vi "tx.vi"(1 "Modulation Parameters In":T2 {"TX Parameters"."TX Sample Rate" items=["4M"]}, 3 "HW parameters in":T3={"Device IP Address"="192.168.11.3", "Active Antenna"="RF1", "Carrier Frequency (Hz)"=2400000000.0, "Gain (dB)"=10.0, "Generation Mode"=enum."single shot"} {"Gain (dB)" format="%.2f"; "Carrier Frequency (Hz)" format="%.2p"}, 5 "Queues in":T1, 7 "error in":errorcluster, 8 "Symbol Energy":dbl=1.0 format="%#_4p") -> (9 "Transmitted IQ Graph":cluster{dbl[], dbl[]}(graph) caption="IQ Graph", 10 "Transmitted Magnitude":dbl[](graph), 11 "Transmitted Constellation Graph":T5(graph) caption="Constellation Graph", 13 "Transmitted Eye Diagram":cluster{"t0":dbl, "dt":dbl, "Y":dbl[]}[](graph) caption="Eye Diagram", 15 "Transmitted I":waveform(dbl)(graph), 16 "Transmitted Phase":dbl[](graph), 17 "Transmitted Q":waveform(dbl)(graph), 19 "Transmitted PSD":dbl[](graph), 20 "HW parameters out":T3={"Device IP Address"="192.168.11.3", "Active Antenna"="RF1", "Carrier Frequency (Hz)"=2400000000.0, "Gain (dB)"=10.0, "Generation Mode"=enum."single shot"} {"Gain (dB)" format="%.2f"; "Carrier Frequency (Hz)" format="%.2p"}, 21 "output complex waveform":cluster{"t0":dbl, "dt":dbl, "Y":cdb[]}, 23 "key bit sequence":u8[](array[numeric]), 25 "data symbols":cdb[](array[numeric]), 27 "error out":errorcluster)   [LabVIEW 2012]
uses:
  EE 497/LABS/SDR/control_type_defs.llb/tx_hw params.ctl
  EE 497/LABS/SDR/control_type_defs.llb/Queues.ctl
panel:
  out "number of data symbols":i32
  in  "TX Graphs":T4(tab)
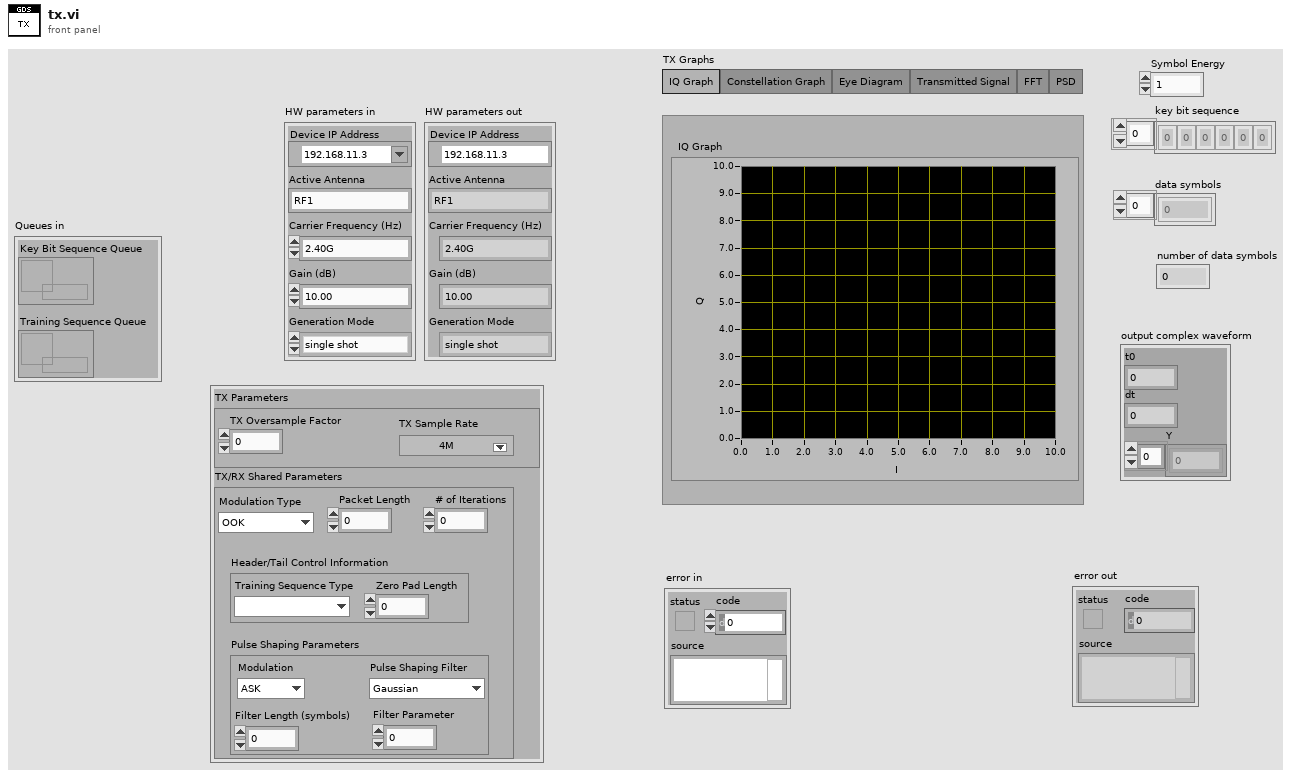
[diagram p1: front panel]
types:
  T1 = typedef "Queues.ctl" = cluster{"Key Bit Sequence Queue":refnum<queue>, "Training Sequence Queue":refnum<queue>}
  T2 = cluster{"TX Parameters":cluster{"TX Oversample Factor":u16, "TX Sample Rate":dbl}, "TX/RX Shared Parameters":cluster{"Modulation Type":enum16{"OOK", "FSK"}, "Packet Length":dbl, "# of Iterations":dbl, "Pulse Shaping Parameters":cluster{"Modulation":enum16{"ASK", "FSK", "PSK", "QAM", "MSK", "PAM"}, "Pulse Shaping Filter":enum16{"Gaussian"}, "Filter Length (symbols)":dbl, "Filter Parameter":dbl}, "Header/Tail Control Information":cluster{"Training Sequence Type":enum16{""}, "Zero Pad Length":dbl}}}
  T3 = typedef "tx_hw params.ctl" = cluster{"Device IP Address":refnum<k15>, "Active Antenna":string, "Carrier Frequency (Hz)":dbl, "Gain (dB)":dbl, "Generation Mode":enum16{"single shot", "simulate", "continuous"}}
  T4 = enum32{"IQ Graph", "Constellation Graph", "Eye Diagram", "Transmitted Signal", "FFT", "PSD"}
  T5 = cluster{"Decimated Array":dbl[], "Decimated Array":dbl[]}[]
  T6 = cluster{"TX Parameters":cluster{"TX Oversample Factor":u16, "TX Sample Rate":dbl}, "TX/RX Shared Parameters":cluster{"Modulation Type":enum16{"OOK", "FSK"}, "Packet Length":u32, "# of Iterations":dbl, "Pulse Shaping Parameters":cluster{"Modulation":enum16{"ASK", "FSK", "PSK", "QAM", "MSK", "PAM"}, "Pulse Shaping Filter":enum16{"Gaussian"}, "Filter Length (symbols)":dbl, "Filter Parameter":dbl}, "Header/Tail Control Information":cluster{"Training Sequence Type":enum16{""}, "Zero Pad Length":dbl}}}
  T7 = cluster{"constellation":dbl[], "oversampled data":dbl[]}[]
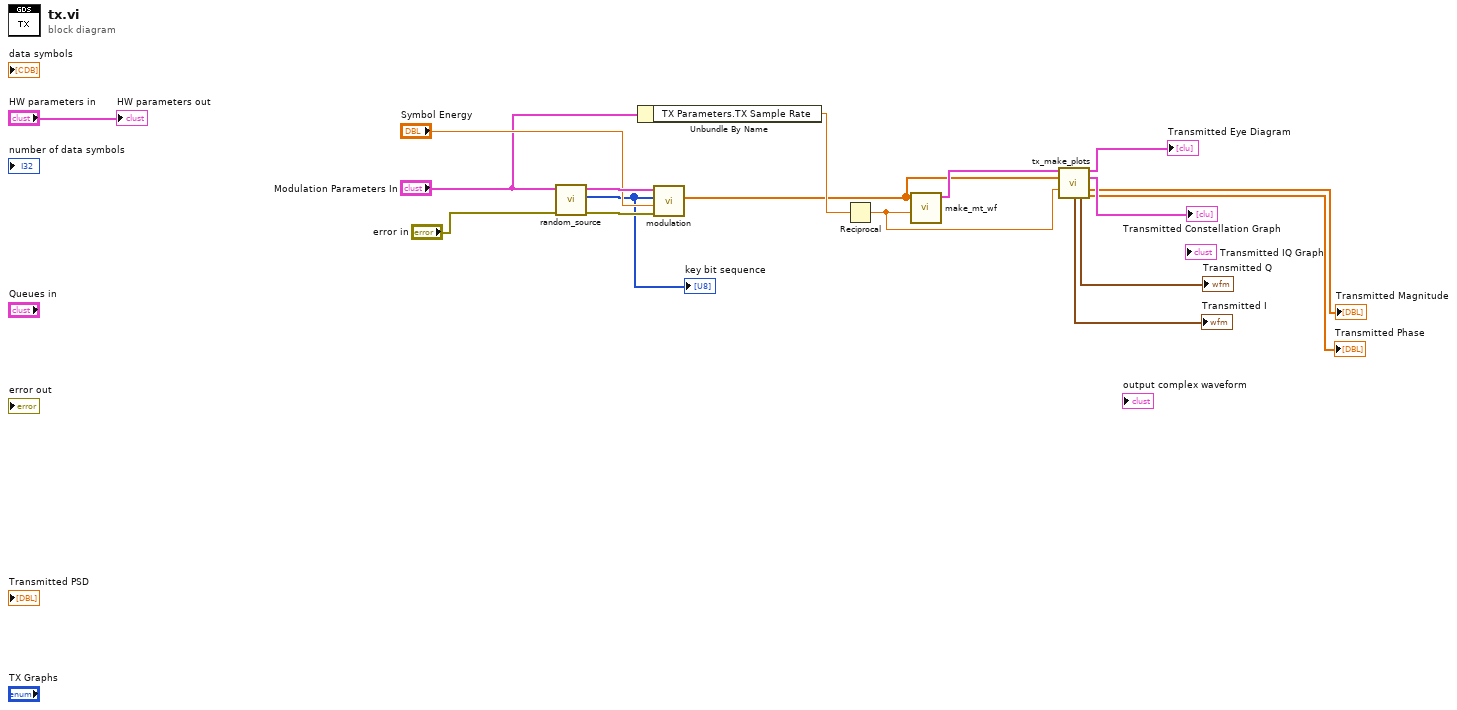
[diagram p0: block diagram]
diagram:
  n1 = call "random_source.vi"("error in (no error)"="error in", "Modulation Parameters In"="Modulation Parameters In") -> ("error out"=w14:errorcluster, "output bit stream"=w1:u8[], "Modulation Parameters Out"=w15:T6)  [unwired: 3 in]
  "key bit sequence" <- w1
  n2 = Unbundle By Name("Modulation Parameters In") -> ("TX Parameters.TX Sample Rate"=w11:dbl)
  n3 = call "modulation.vi"("error in"=w14, "Symbol Energy"="Symbol Energy", "input bit stream"=w1, "Modulation Parameters In"=w15) -> ("Output Symbols"=w9:cdb[])  [unwired: 5 in, 2 out]
  n4 = Reciprocal(x=w11) -> (1/x=w2:dbl)
  n5 = call "make_mt_wf.vi"("dt"=w2, "Y"=w9) -> ("output MT waveform"=w10:cluster{"t0":dbl, "dt":dbl, "Y":cdb[]})  [unwired: 9 in]
  n6 = call "tx_make_plots.vi"("waveform"=w10, "Y"=w9, "symbol rate (Hz)"=w2) -> ("eye diagram"=→"Transmitted Eye Diagram":cluster{"t0":dbl, "dt":dbl, "Y":dbl[]}[], "constellation graph"=→"Transmitted Constellation Graph":T7, "r"=→"Transmitted Magnitude":dbl[], "I component"=→"Transmitted I":waveform(dbl), "Q component"=→"Transmitted Q":waveform(dbl), "theta"=→"Transmitted Phase":dbl[])  [unwired: 6 in, 1 out]
  "HW parameters out" <- "HW parameters in"
